vi "CoolLED_by_Functions_2.vi"(8 "error in (no error)":errorcluster, 11 "Message Queue":refnum<queue>) -> (0 "error out":errorcluster)   [LabVIEW 2025]
uses:
  LABVIEW_QCM_v2.0/Labview_code/QCM_2.0_LV_1.2/QMH/Message Queue/Message Cluster.ctl
  LABVIEW_QCM_v2.0/Labview_code/QCM_2.0_LV_1.2/QMH/Message Queue/Message Queue.lvlib
panel:
  out "Presets":bool
  out "Settings":bool
  out "Store":bool
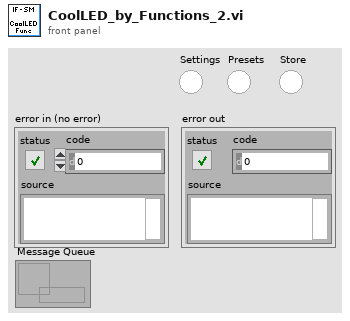
[diagram p1: front panel]
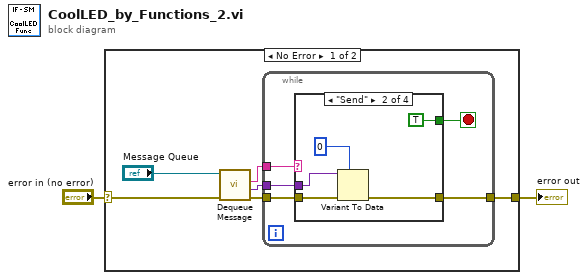
[diagram p0: block diagram]
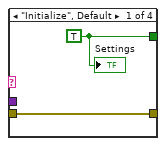
[diagram p2: hidden frame]
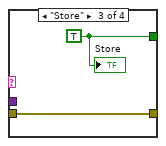
[diagram p3: hidden frame]
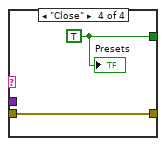
[diagram p4: hidden frame]
diagram:
  n1 = case shown="No Error" "error in (no error)" {
    selector: "error in (no error)" -> [w7 w25]
    tunnel: [w3 w25] -> w2
    frame No Error {
      n2 = call "Dequeue Message.vi"("error in (no error)"=w7, "Message Queue"="Message Queue") -> ("error out"=w5:errorcluster, "Message Data"=w4:variant, "Message"=w6:string)  [unwired: 6 in, 1 out]
      n3 = while {
        tunnel: w6 -> [w12]
        tunnel: w5 -> [w11]
        tunnel: w4 -> [w10]
        tunnel: [w9] -> w3
        stop <- w13 stop-if-true
        n4 = case shown="\"Send\"" w12 {
          tunnel: [w15 TRUE w22 w24] -> w13
          tunnel: w11 -> [w14 w19 w21 w23]
          tunnel: w10 -> [_ w18 _ _]
          tunnel: [w14 w16 w21 w23] -> w9
          frame "Initialize", Default {
            w15 = TRUE
            "Settings" <- w15
          }
          frame "Send" {
            n5 = Variant To Data(error in=w19, type=u8 0, Variant=w18) -> (error out=w16:errorcluster)  [unwired: 1 out]
          }
          frame "Store" {
            w22 = TRUE
            "Store" <- w22
          }
          frame "Close" {
            w24 = TRUE
            "Presets" <- w24
          }
        }
      }
    }
    frame Error {
    }
  }
  "error out" <- w2
